vi "Agilent 415X Series Dual Source Sweep Display.vi"() -> ()   [LabVIEW 2016]
doc: "This VI is an example of how HP415xA subVIs can be used programmatically for a SWEEP mode operation.\n\nIt will initialize and close the instrument and driver."
uses:
  Agilent 415X Series.lvlib
panel:
  out "graphic display":cluster{dbl[], dbl[]}[](graph)
  out "Y":dbl[](array[numeric]) format="%^.3e"
  in  "Y name":string="I3"
  out "X":dbl[](array[numeric]) format="%^.3e"
  in  "X name":string="V3"
  in  "secondary source":cluster{"start":dbl, "step size":dbl}={"start"=2e-05, "step size"=2e-05} {"step size" format="%^.4e"; "start" format="%^.4e"}
  in  "primary source":T1={"sweep mode"=FALSE, "sweep spacing\n(linear: 0)"=0, "start"=0.0, "stop"=1.0, "step (linear only)"=0.01} {"step (linear only)" format="%^.4e"; "stop" format="%^.4e"; "start" format="%^.4e"; "sweep spacing\n(linear: 0)" items=["linear", "log 10", "log 25", "log 50"]}
  in  "wait time parameter":dbl=1.0 format="%.1f"
  in  "integration time":i32(slide) scale=0.0..2.0
  in  "VSU2 source":dbl format="%.4f"
  in  "VSU1 source":dbl format="%.4f"
  in  "SMU4 source":dbl format="%.4f"
  # "(c) 2005-2015 National Instruments.  ALL RIGHTS RESERVED."
  # "Semiconductor Parameter Analyzer 4155A/4156A"
  # "channel definition"
  # "Unit \n  SMU1 \n  SMU2\n  SMU3\n  SMU4\n  VSU1\n  VSU2\n  VMU1     \n  VMU2"
  # "V Name\n  V1\n  V2\n  V3\n  V4\n  VSU1\n  VSU2\n  VMU1\n  VMU2"
  # "I Name\n  I1\n  I2\n  I3\n  I4\n  --\n  --\n  --\n  --"
  # "Mode \n COM\n I\n V\n V\n V\n V\n --\n --"
  # "Function\n constant \n secondary sweep source \n primary sweep source\n constant                       V\n constant                       V\n constant                       V\n       -\n       -"
  # "Range\n limited (1nA) \n auto\n limited (1nA)\n limited (1nA)\n auto\n auto\n   --\n   --"
  # "* total steps = 5"
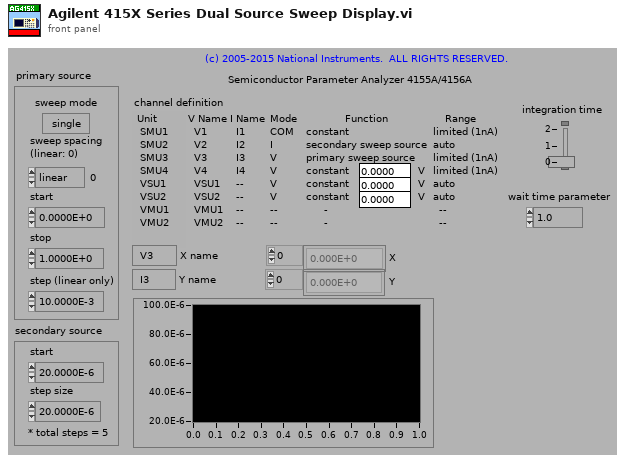
[diagram p1: front panel]
types:
  T1 = cluster{"sweep mode":bool, "sweep spacing\n(linear: 0)":u16, "start":dbl, "stop":dbl, "step (linear only)":dbl}
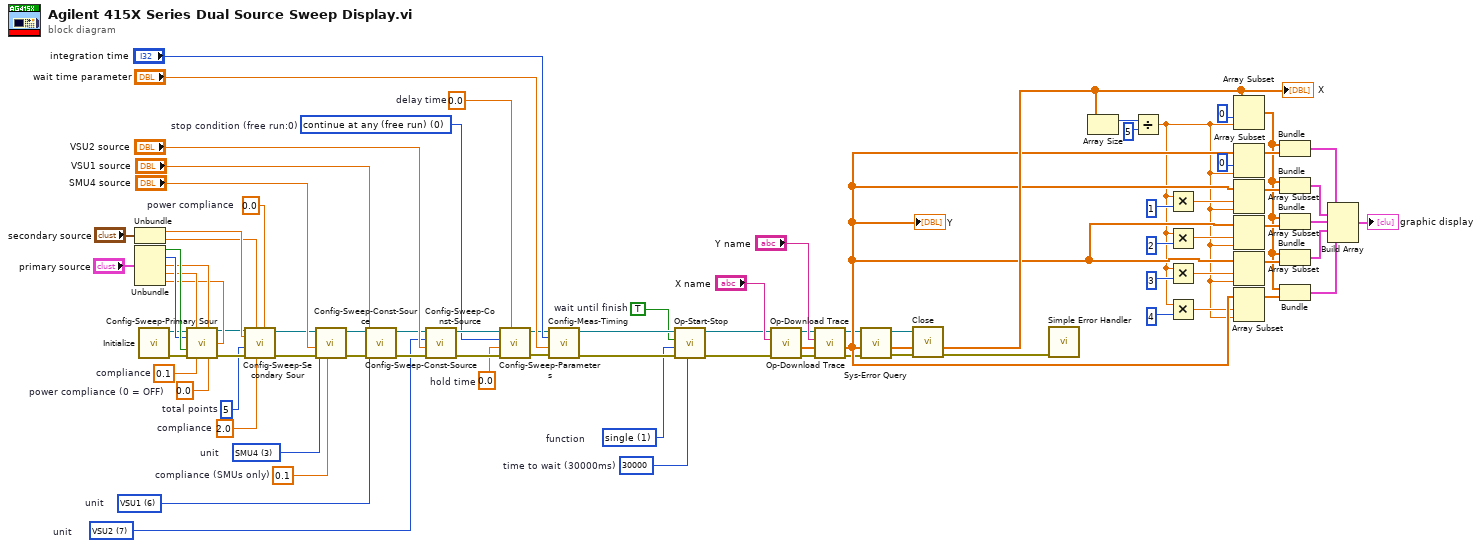
[diagram p0: block diagram]
diagram:
  w1 = u8 0 items=["continue at any (free run)", "stop at any abnorm", "stop at compliance"]  # stop condition (free run:0)
  w2 = 5  # total points
  w3 = 0.0  # hold time
  w4 = 0.0  # delay time
  w5 = 1 items=["stop  ", "single  ", "single-append  ", "stress start  ", "continuous  ", "standby on  ", "standby off  ", "zero  "]  # function
  w6 = u16 7 items=["SMU 1", "SMU2", "SMU3", "SMU4", "SMU5", "SMU6", "VSU1", "VSU2"]  # unit
  w7 = u16 6 items=["SMU 1", "SMU2", "SMU3", "SMU4", "SMU5", "SMU6", "VSU1", "VSU2"]  # unit
  w8 = 0.1  # compliance (SMUs only)
  w9 = u16 3 items=["SMU 1", "SMU2", "SMU3", "SMU4", "SMU5", "SMU6", "VSU1", "VSU2"]  # unit
  w10 = 0.0  # power compliance
  w11 = 2.0  # compliance
  w12 = 0.0  # power compliance (0 = OFF)
  w13 = 0.1  # compliance
  w14 = TRUE  # wait until finish
  w30 = u32 30000  # time to wait (30000ms)
  n1 = Unbundle("secondary source") -> ("start"=w75:dbl, "step size"=w29:dbl)
  n2 = Unbundle("primary source") -> ("sweep mode"=w82:bool, "sweep spacing\n(linear: 0)"=w81:u16, "start"=w80:dbl, "stop"=w79:dbl, "step (linear only)"=w78:dbl)
  n3 = call "Initialize.vi"() -> ("error out"=w33:errorcluster, "VISA resource name out"=w32:refnum<visa-resource-name>)  [unwired: 10 in]
  n4 = call "Config-Sweep-Primary Sour.vi"("VISA session"=w32, "stop"=w79, "start"=w80, "sweep spacing (linear: 0)"=w81, "step (linear only)"=w78, "sweep mode"=w82, "error in (no error)"=w33, "compliance"=w13, "power compliance (0 = OFF)"=w12) -> ("VISA resource name out"=w26:refnum<visa-resource-name>, "error out"=w77:errorcluster)  [unwired: 5 in]
  n5 = call "Config-Sweep-Secondary Sour.vi"("power compliance (0 = OFF)"=w10, "compliance"=w11, "step"=w29, "error in (no error)"=w77, "total points"=w2, "start"=w75, "VISA session"=w26) -> ("error out"=w74:errorcluster, "VISA resource name out"=w25:refnum<visa-resource-name>)  [unwired: 3 in]
  n6 = call "Config-Sweep-Const-Source.vi"("compliance (SMUs only)"=w8, "error in (no error)"=w74, "source (V or A)"="SMU4 source", "unit (SMU1:0)"=w9, "VISA session"=w25) -> ("error out"=w72:errorcluster, "VISA resource name out"=w24:refnum<visa-resource-name>)  [unwired: 5 in]
  n7 = call "Config-Sweep-Const-Source.vi"("error in (no error)"=w72, "source (V or A)"="VSU1 source", "unit (SMU1:0)"=w7, "VISA session"=w24) -> ("error out"=w69:errorcluster, "VISA resource name out"=w23:refnum<visa-resource-name>)  [unwired: 6 in]
  n8 = call "Config-Sweep-Const-Source.vi"("error in (no error)"=w69, "source (V or A)"="VSU2 source", "unit (SMU1:0)"=w6, "VISA session"=w23) -> ("error out"=w68:errorcluster, "VISA resource name out"=w22:refnum<visa-resource-name>)  [unwired: 6 in]
  n9 = call "Config-Sweep-Parameters.vi"("delay time (sec)"=w4, "error in (no error)"=w68, "hold time (sec)"=w3, "stop condition (free run:0)"=w1, "VISA session"=w22) -> ("error out"=w67:errorcluster, "VISA resource name out"=w21:refnum<visa-resource-name>)  [unwired: 5 in]
  n10 = call "Config-Meas-Timing.vi"("error in (no error)"=w67, "wait time parameter"="wait time parameter", "integration time"="integration time", "VISA session"=w21) -> ("error out"=w64:errorcluster, "VISA resource name out"=w20:refnum<visa-resource-name>)  [unwired: 6 in]
  n11 = call "Op-Start-Stop.vi"("time to wait (30000ms)"=w30, "error in (no error)"=w64, "function (stop:0)"=w5, "wait until finish"=w14, "VISA resource name"=w20) -> ("error out"=w63:errorcluster, "VISA resource name out"=w19:refnum<visa-resource-name>)  [unwired: 5 in]
  n12 = call "Op-Download Trace.vi"("error in (no error)"=w63, "trace (variable) name"="X name", "VISA session"=w19) -> ("error out"=w62:errorcluster, "trace"=w58:dbl[], "VISA resource name out"=w18:refnum<visa-resource-name>)  [unwired: 6 in]
  "X" <- w58
  n13 = call "Op-Download Trace.vi"("error in (no error)"=w62, "trace (variable) name"="Y name", "VISA session"=w18) -> ("error out"=w46:errorcluster, "trace"=w56:dbl[], "VISA resource name out"=w17:refnum<visa-resource-name>)  [unwired: 6 in]
  "Y" <- w56
  n14 = call "Sys-Error Query.vi"("error in (no error)"=w46, "VISA session"=w17) -> ("error out"=w31:errorcluster, "VISA resource name out"=w16:refnum<visa-resource-name>)  [unwired: 7 in, 1 out]
  n15 = call "Close.vi"("error in (no error)"=w31, "VISA resource name"=w16) -> ("error out"=w15:errorcluster)  [unwired: 9 in]
  n16 = call <vilib>:"Simple Error Handler.vi"("error in (no error)"=w15) -> ()  [unwired: 4 in, 5 out]
  n17 = Array Size(array=w58) -> (size(s)=w61:i32)
  n18 = Divide(x=w61, y=5) -> (x/y=w47:dbl)
  n19 = Multiply(x=w47, y=1) -> (x*y=w54:dbl)
  n20 = Multiply(x=w47, y=2) -> (x*y=w48:dbl)
  n21 = Multiply(x=w47, y=3) -> (x*y=w49:dbl)
  n22 = Multiply(x=w47, y=4) -> (x*y=w50:dbl)
  n23 = Array Subset(array=w58, index=0, length=w47) -> (w40:dbl[])
  n24 = Array Subset(array=w56, index=0, length=w47) -> (w45:dbl[])
  n25 = Array Subset(array=w56, index=w54, length=w47) -> (w44:dbl[])
  n26 = Array Subset(array=w56, index=w48, length=w47) -> (w43:dbl[])
  n27 = Array Subset(array=w56, index=w49, length=w47) -> (w42:dbl[])
  n28 = Array Subset(array=w56, index=w50, length=w47) -> (w41:dbl[])
  n29 = Bundle(w40, w45) -> (w39:cluster{dbl[], dbl[]})  [unwired: 1 in]
  n30 = Bundle(w40, w44) -> (w38:cluster{dbl[], dbl[]})  [unwired: 1 in]
  n31 = Bundle(w40, w43) -> (w37:cluster{dbl[], dbl[]})  [unwired: 1 in]
  n32 = Bundle(w40, w42) -> (w36:cluster{dbl[], dbl[]})  [unwired: 1 in]
  n33 = Bundle(w40, w41) -> (w35:cluster{dbl[], dbl[]})  [unwired: 1 in]
  n34 = Build Array(w39, w38, w37, w36, w35) -> (→"graphic display":cluster{dbl[], dbl[]}[])
